vi "closeConnection.vi"(8 "error in (no error)":errorcluster, 10 "quit python":bool=TRUE, 11 "LabVIEW-Python-Interface in":refnum<class "PyLVi.lvclass">) -> (0 "error out":errorcluster, 3 "LabVIEW-Python-Interface out":refnum<class "PyLVi.lvclass">)   [LabVIEW 2016, in "PyLVi.lvlib" / "PyLVi.lvclass"]
uses:
  PyLVi.lvclass
  PyLVi.lvclass/PyLVi.ctl
  <vilib>/addons/zeromq/zmq_socket.lvclass
  <vilib>/addons/zeromq/zmq_context.lvclass
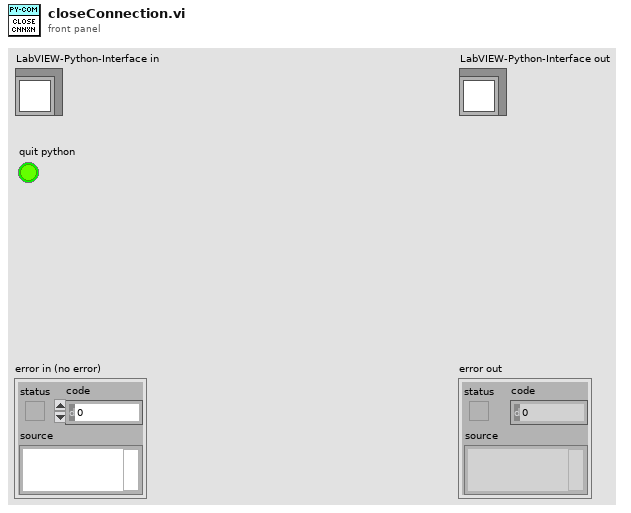
[diagram p1: front panel]
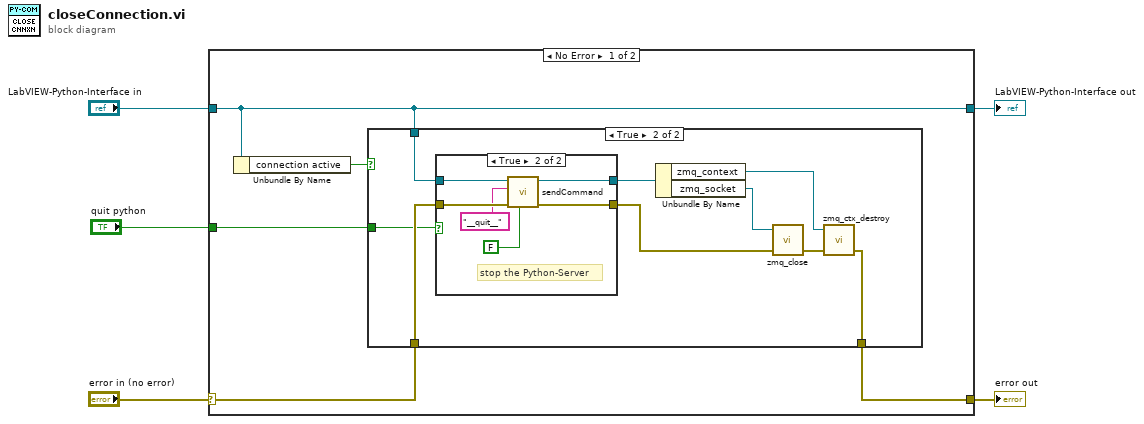
[diagram p0: block diagram]
diagram:
  n1 = case shown="No Error" "error in (no error)" {
    selector: "error in (no error)" -> [w9 w30]
    tunnel: [w10 w30] -> w4
    tunnel: [w8 w29] -> w2
    tunnel: "LabVIEW-Python-Interface in" -> [w8 w29]
    tunnel: "quit python" -> [w6 _]
    frame No Error {
      n2 = Unbundle By Name(w8) -> ("connection active"=w7:bool)
      n3 = case shown="True" w7 {
        tunnel: [w11 w19] -> w10
        tunnel: w9 -> [w11 w15]
        tunnel: w8 -> [_ w13]
        tunnel: w6 -> [_ w12]
        frame False {
        }
        frame True {
          n4 = case shown="True" w12 {
            tunnel: [w22 w28] -> w16
            tunnel: w15 -> [w21 w27]
            tunnel: [w21 w26] -> w14
            tunnel: w13 -> [w22 w23]
            frame False {
            }
            frame True {
              # "stop the Python-Server"
              n5 = call "sendCommand.vi"("Wait for response (T)"=FALSE, "error in (no error)"=w27, "command"="__quit__", "LabVIEW-Python-Interface in"=w23) -> ("error out"=w26:errorcluster, "LabVIEW-Python-Interface out"=w28:refnum<class "PyLVi.lvclass">)  [unwired: 4 in, 2 out]
            }
          }
          n6 = Unbundle By Name(w16) -> ("zmq_context"=w17:refnum<class "zmq_context.lvclass">, "zmq_socket"=w18:refnum<class "zmq_socket.lvclass">)
          n7 = call <vilib>:"zmq_close.vi"("error in"=w14, "socket"=w18) -> ("error out"=w20:errorcluster)  [unwired: 3 in]
          n8 = call <vilib>:"zmq_ctx_destroy.vi"("error in"=w20, "context in"=w17) -> ("error out"=w19:errorcluster)  [unwired: 3 in]
        }
      }
    }
    frame Error {
    }
  }
  "error out" <- w4
  "LabVIEW-Python-Interface out" <- w2
